vi "Function.vi"(8 "error in (no error)":errorcluster, 10 "Waveform":waveform(dbl), 11 "Two Terminal in":refnum<class "Invert_WFM.lvclass">) -> (0 "error out":errorcluster, 2 "Result":waveform(dbl), 3 "Two Terminal out":refnum<class "Invert_WFM.lvclass">)   [LabVIEW 2021, in "Invert_WFM.lvclass"]
uses:
  Invert_WFM.lvclass
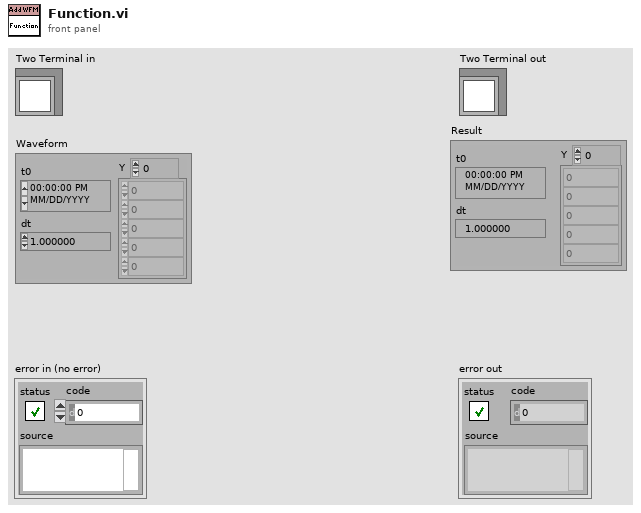
[diagram p1: front panel]
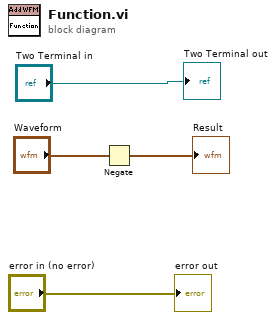
[diagram p0: block diagram]
diagram:
  n1 = Negate(x="Waveform") -> (-x=→"Result":waveform(dbl))
  "error out" <- "error in (no error)"
  "Two Terminal out" <- "Two Terminal in"
